vi "MATLAB-LabView 1.vi"() -> ()   [LabVIEW 2015]
panel:
  out "Waveform Graph":dbl[](graph)
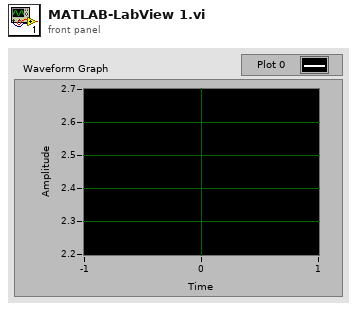
[diagram p1: front panel]
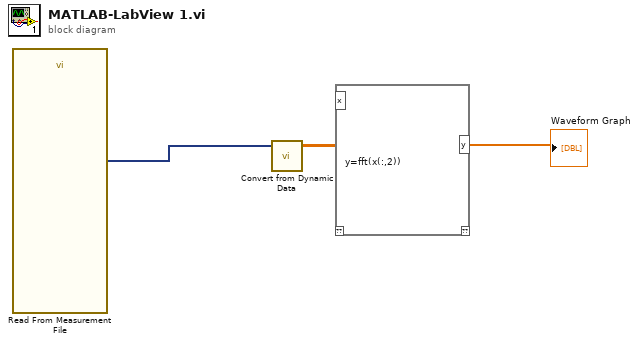
[diagram p0: block diagram]
diagram:
  n1 = call "Read From Measurement File"() -> ("Signals"=w2:dynamicdata)  [unwired: 6 in, 5 out]
  n2 = call "Convert from Dynamic Data"("Dynamic Data Type"=w2) -> ("Array"=w1:dbl[][])  [unwired: 3 in]
  n3 = script code="y=fft(x(:,2))"("x"=w1) -> ("y"=→"Waveform Graph":dbl[])  [unwired: 1 in, 1 out]
